vi "UI - Initiate Connection.vi"(8 "error in (no error)":errorcluster, 10 "Controller Address":string, 11 "Message Queue":refnum<queue>) -> (0 "error out":errorcluster, 1 "Connected?":bool, 3 "dup Message Queue":refnum<queue>)   [LabVIEW 2015]
uses:
  Message Queue/Message Cluster.ctl
  controls/Variable References.ctl
  Globals/Global - Configuration Options.vi
  Globals/Global - UI Stream and Variable Connections.vi
  Message Queue/Message Queue.lvlib
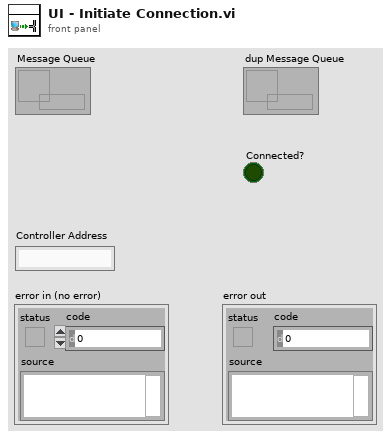
[diagram p1: front panel]
types:
  T1 = typedef "Message Queue.lvlib/Message Cluster.ctl" = cluster{"Message":string, "Message Data":variant}
  T2 = typedef "Variable References.ctl" = cluster{"CPU Usage":refnum<k21>, "Contiguous Memory":refnum<k21>, "Actual Loop Period":refnum<k21>, "Buffer Backlog":refnum<k21>, "Drive Space":refnum<k21>, "Number of Data Files":refnum<k21>, "System Time":refnum<k21>}
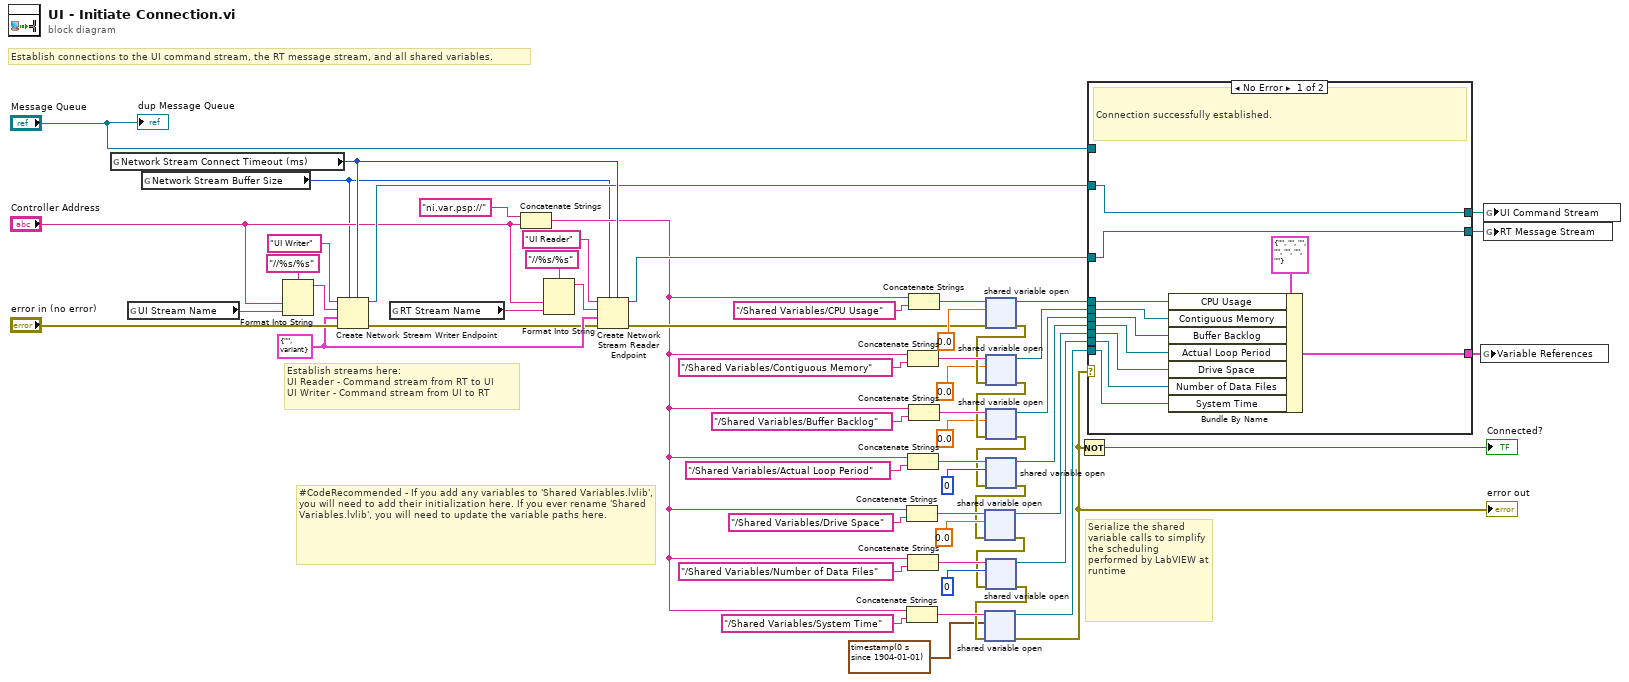
[diagram p0: block diagram]
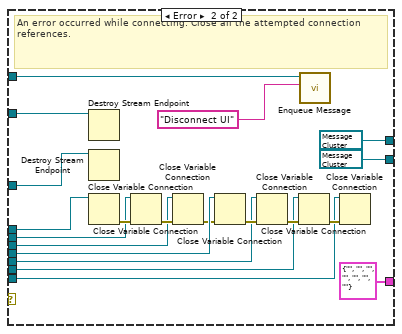
[diagram p2: hidden frame]
diagram:
  w49 = T1 {"Message"="", "Message Data"=variant} ("Message Cluster")
  # "Establish connections to the UI command stream, the RT message stream, and all shared variables."
  # "#CodeRecommended - If you add any variables to 'Shared Variables.lvlib', you will need to add their initialization here. If you ever rename 'Shared Variables.lvlib', you will need to update the variable paths here."
  # "Establish streams here:\nUI Reader - Command stream from RT to UI\nUI Writer - Command stream from UI to RT"
  # "Serialize the shared variable calls to simplify the scheduling performed by LabVIEW at runtime"
  n1 = global read "Global - Configuration Options.vi" "Network Stream Connect Timeout (ms)"() -> (w47:i32)
  n2 = global read "Global - Configuration Options.vi" "UI Stream Name"() -> (w54:string)
  n3 = global read "Global - Configuration Options.vi" "Network Stream Buffer Size"() -> (w2:i32)
  n4 = Format Into String(format string="//%s/%s", "Controller Address", w54) -> (resulting string=w53:string)  [unwired: 2 in, 1 out]
  n5 = Create Network Stream Writer Endpoint(5:w47, 7:w2, 8:"error in (no error)", 9:w49, 10:w53, 11:"UI Writer" ("reader name")) -> (0:w48:errorcluster, 3:w27:refnum<k21>)  [unwired: 1 in]
  n6 = global read "Global - Configuration Options.vi" "RT Stream Name"() -> (w57:string)
  n7 = Concatenate Strings("ni.var.psp://", "Controller Address") -> (w6:string)
  n8 = Format Into String(format string="//%s/%s", "Controller Address", w57) -> (resulting string=w56:string)  [unwired: 2 in, 1 out]
  n9 = Create Network Stream Reader Endpoint(5:w47, 7:w2, 8:w48, 9:w49, 10:w56, 11:"UI Reader" ("writer name")) -> (0:w44:errorcluster, 3:w28:refnum<k21>)  [unwired: 1 in]
  n10 = Concatenate Strings(w6, "/Shared Variables/Drive Space") -> (w19:string)
  n11 = Concatenate Strings(w6, "/Shared Variables/System Time") -> (w10:string)
  n12 = Concatenate Strings(w6, "/Shared Variables/Contiguous Memory") -> (w40:string)
  n13 = Concatenate Strings(w6, "/Shared Variables/Actual Loop Period") -> (w36:string)
  n14 = Concatenate Strings(w6, "/Shared Variables/Number of Data Files") -> (w13:string)
  n15 = Concatenate Strings(w6, "/Shared Variables/CPU Usage") -> (w43:string)
  n16 = Concatenate Strings(w6, "/Shared Variables/Buffer Backlog") -> (w39:string)
  n17 = shared-variable-open(w43, w44, 0.0) -> (w32:refnum<k21>, w34:errorcluster)  [unwired: 1 in]
  n18 = shared-variable-open(w40, w34, 0.0) -> (w31:refnum<k21>, w33:errorcluster)  [unwired: 1 in]
  n19 = shared-variable-open(w39, w33, 0.0) -> (w30:refnum<k21>, w23:errorcluster)  [unwired: 1 in]
  n20 = shared-variable-open(w36, w23, u32 0) -> (w29:refnum<k21>, w18:errorcluster)  [unwired: 1 in]
  n21 = shared-variable-open(w19, w18, 0.0) -> (w17:refnum<k21>, w12:errorcluster)  [unwired: 1 in]
  n22 = shared-variable-open(w13, w12, u32 0) -> (w11:refnum<k21>, w9:errorcluster)  [unwired: 1 in]
  n23 = shared-variable-open(w10, w9, timestamp(0 s since 1904-01-01) ("time stamp")) -> (w7:refnum<k21>, w8:errorcluster)  [unwired: 1 in]
  "error out" <- w8
  n24 = Not(x=w8) -> (.not. x?=→"Connected?":bool)
  n25 = case shown="No Error" w8 {
    tunnel: w32 -> [w69 w86]
    tunnel: w31 -> [w68 w83]
    tunnel: w30 -> [w67 w84]
    tunnel: w29 -> [w66 w85]
    tunnel: w28 -> [w63 w89]
    tunnel: w27 -> [w64 w90]
    tunnel: [w65 T2 {"CPU Usage"="", "Contiguous Memory"="", "Actual Loop Period"="", "Buffer Backlog"="", "Drive Space"="", "Number of Data Files"="", "System Time"=""} ("Variable References")] -> w26
    tunnel: [w64 refnum<k21> refnum] -> w25
    tunnel: [w63 refnum<k21> refnum] -> w24
    tunnel: w17 -> [w62 w79]
    tunnel: w11 -> [w61 w77]
    tunnel: w7 -> [w60 w75]
    tunnel: "Message Queue" -> [_ w72]
    frame No Error {
      # "Connection successfully established."
      n26 = Bundle By Name(cluster=T2 {"CPU Usage"="", "Contiguous Memory"="", "Actual Loop Period"="", "Buffer Backlog"="", "Drive Space"="", "Number of Data Files"="", "System Time"=""} ("Variable References"), "CPU Usage"=w69, "Contiguous Memory"=w68, "Buffer Backlog"=w67, "Actual Loop Period"=w66, "Drive Space"=w62, "Number of Data Files"=w61, "System Time"=w60) -> (w65:T2)
    }
    frame Error {
      # "An error occurred while connecting. Close all the attempted connection references."
      n27 = Destroy Stream Endpoint(11:w90) -> ()  [unwired: 1 in, 1 out]
      n28 = Destroy Stream Endpoint(11:w89) -> ()  [unwired: 1 in, 1 out]
      n29 = Close Variable Connection(11:w86) -> (0:w87:errorcluster)  [unwired: 1 in]
      n30 = Close Variable Connection(8:w87, 11:w83) -> (0:w88:errorcluster)
      n31 = Close Variable Connection(8:w88, 11:w84) -> (0:w81:errorcluster)
      n32 = Close Variable Connection(8:w81, 11:w85) -> (0:w80:errorcluster)
      n33 = Close Variable Connection(8:w80, 11:w79) -> (0:w78:errorcluster)
      n34 = Close Variable Connection(8:w78, 11:w77) -> (0:w76:errorcluster)
      n35 = call "Enqueue Message.vi"("Message"="Disconnect UI", "Message Queue"=w72) -> ()  [unwired: 8 in, 2 out]
      n36 = Close Variable Connection(8:w76, 11:w75) -> ()  [unwired: 1 out]
    }
  }
  n37 = global write "Global - UI Stream and Variable Connections.vi" "Variable References"(w26) -> ()
  n38 = global write "Global - UI Stream and Variable Connections.vi" "UI Command Stream"(w25) -> ()
  n39 = global write "Global - UI Stream and Variable Connections.vi" "RT Message Stream"(w24) -> ()
  "dup Message Queue" <- "Message Queue"
